vi "Less String.vi"(11 "Input String":string) -> (3 "Out String":string)   [LabVIEW 2024]
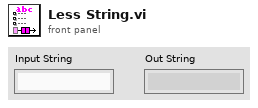
[diagram p1: front panel]
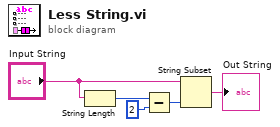
[diagram p0: block diagram]
diagram:
  n1 = String Length(string="Input String") -> (length=w1:i32)
  n2 = Subtract(x=w1, y=2) -> (x-y=w3:i32)
  n3 = String Subset(string="Input String", length (rest)=w3) -> (substring=→"Out String":string)  [unwired: 1 in]
